vi "sinh.vi"(8 "# points":u32, 9 "B":dbl, 10 "Amp":dbl[](array[numeric]), 11 "T":dbl[](array[numeric])) -> (1 "mass":dbl, 2 "Amp":dbl[](array[numeric]), 3 "T":dbl[](array[numeric]))   [LabVIEW 2015]
uses:
  <vilib>/Analysis/baseanly.llb/Mean (DBL).vi
  <vilib>/Analysis/NI_AALBase.lvlib
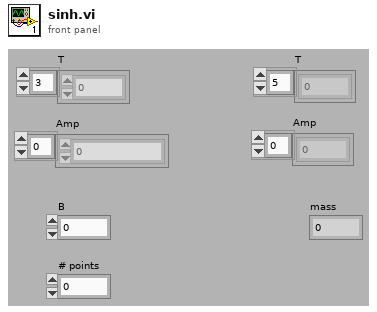
[diagram p1: front panel]
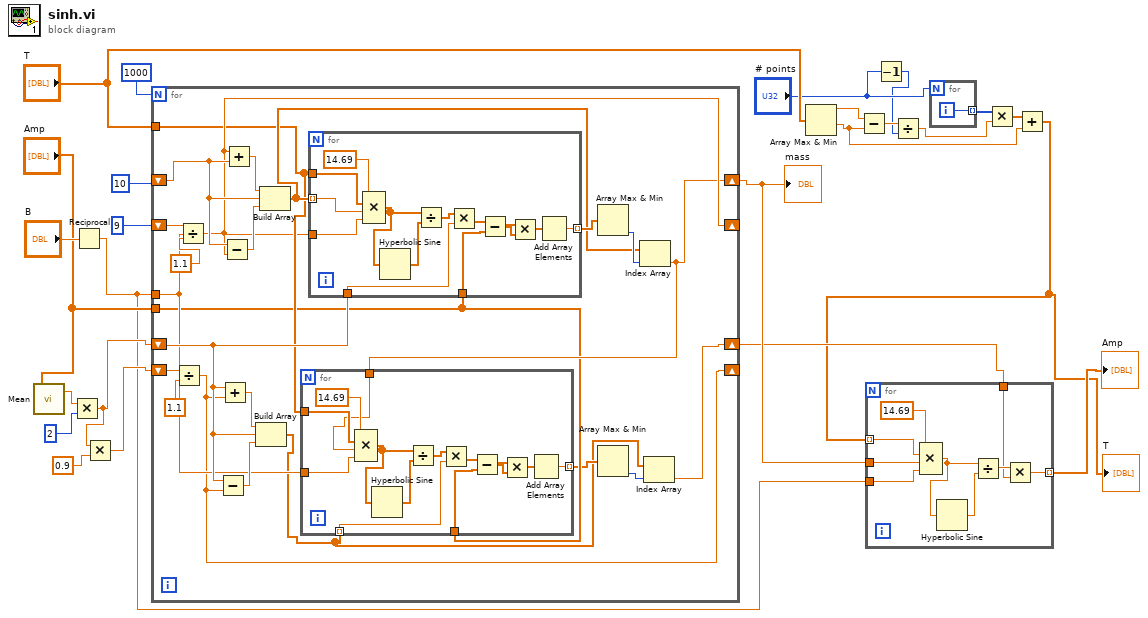
[diagram p0: block diagram]
diagram:
  n1 = call-poly <vilib>:"Mean.vi"("X"="Amp") -> ("mean"=w17:dbl)  [unwired: 1 out]
  n2 = Multiply(x=w17, y=2) -> (x*y=w18:dbl)
  n3 = Reciprocal(x="B") -> (1/x=w4:dbl)
  n4 = Multiply(x=w18, y=0.9) -> (x*y=w16:dbl)
  n5 = for {
    N: 1000 -> [_]
    shift-right: [w31] -> w5
    shift-left: 10 -> [w44]
    shift-right: [w39] -> _
    shift-left: 9 -> [w47]
    tunnel: "T" -> [w33]
    tunnel: [w32] -> _ mode=indexing
    tunnel: w4 -> [w32]
    shift-right: [w26] -> w3
    shift-left: w18 -> [w36]
    shift-right: [w25] -> _
    shift-left: w16 -> [w35]
    tunnel: "Amp" -> [w30]
    n6 = Divide(x=w35, y=1.1) -> (x/y=w25:dbl)
    n7 = Divide(x=w47, y=1.1) -> (x/y=w39:dbl)
    n8 = Subtract(x=w36, y=w25) -> (x-y=w37:dbl)
    n9 = Add(x=w36, y=w25) -> (x+y=w38:dbl)
    n10 = Subtract(x=w44, y=w39) -> (x-y=w43:dbl)
    n11 = Add(x=w39, y=w44) -> (x+y=w45:dbl)
    n12 = Build Array(w38, w36, w37) -> (w27:dbl[])
    n13 = Build Array(w45, w44, w43) -> (w40:dbl[])
    n14 = for {
      tunnel: w40 -> [w71] mode=indexing
      tunnel: w33 -> [w72]
      tunnel: w32 -> [w70]
      tunnel: w36 -> [w66]
      tunnel: w30 -> [w64]
      tunnel: [w61] -> w42 mode=indexing
      n15 = Compound Arithmetic op=MULTIPLY(14.69, w72, w71, w70) -> (w69:dbl[])
      n16 = Hyperbolic Sine(1:w69) -> (0:w68:dbl[])
      n17 = Divide(x=w69, y=w68) -> (x/y=w67:dbl[])
      n18 = Multiply(x=w67, y=w66) -> (x*y=w65:dbl[])
      n19 = Subtract(x=w65, y=w64) -> (x-y=w63:dbl[])
      n20 = Multiply(x=w63, y=w63) -> (x*y=w62:dbl[])
      n21 = Add Array Elements(numeric array=w62) -> (sum=w61:dbl)
    }
    n22 = Array Max & Min(array=w42) -> (min index (indices)=w41:i32)  [unwired: 3 out]
    n23 = Index Array(array=w40, index=w41) -> (element=w31:dbl)
    n24 = for {
      tunnel: w33 -> [w59]
      tunnel: w32 -> [w58]
      tunnel: w27 -> [w54] mode=indexing
      tunnel: w30 -> [w52]
      tunnel: [w49] -> w29 mode=indexing
      tunnel: w31 -> [w48]
      n25 = Compound Arithmetic op=MULTIPLY(14.69, w59, w48, w58) -> (w57:dbl[])
      n26 = Hyperbolic Sine(1:w57) -> (0:w56:dbl[])
      n27 = Divide(x=w57, y=w56) -> (x/y=w55:dbl[])
      n28 = Multiply(x=w55, y=w54) -> (x*y=w53:dbl[])
      n29 = Subtract(x=w53, y=w52) -> (x-y=w51:dbl[])
      n30 = Multiply(x=w51, y=w51) -> (x*y=w50:dbl[])
      n31 = Add Array Elements(numeric array=w50) -> (sum=w49:dbl)
    }
    n32 = Array Max & Min(array=w29) -> (min index (indices)=w28:i32)  [unwired: 3 out]
    n33 = Index Array(array=w27, index=w28) -> (element=w26:dbl)
  }
  "mass" <- w5
  n34 = Array Max & Min(array="T") -> (max value=w13:dbl, min value=w6:dbl)  [unwired: 2 out]
  n35 = Subtract(x=w13, y=w6) -> (x-y=w11:dbl)
  n36 = Decrement(x="# points") -> (x-1=w10:u32)
  n37 = Divide(x=w11, y=w10) -> (x/y=w8:dbl)
  n38 = for {
    N: "# points" -> [_]
    tunnel: [w74] -> w9 mode=indexing
    i -> [w74]
  }
  n39 = Multiply(x=w9, y=w8) -> (x*y=w7:dbl[])
  n40 = Add(x=w7, y=w6) -> (x+y=w1:dbl[])
  "T" <- w1
  n41 = for {
    tunnel: w1 -> [w80] mode=indexing
    tunnel: w5 -> [w79]
    tunnel: w4 -> [w78]
    tunnel: w3 -> [w76]
    tunnel: [w75] -> w2 mode=indexing
    n42 = Compound Arithmetic op=MULTIPLY(14.69, w80, w79, w78) -> (w82:dbl)
    n43 = Hyperbolic Sine(1:w82) -> (0:w81:dbl)
    n44 = Divide(x=w82, y=w81) -> (x/y=w77:dbl)
    n45 = Multiply(x=w77, y=w76) -> (x*y=w75:dbl)
  }
  "Amp" <- w2
